vi "manuele bediening.vi"   [LabVIEW 2019]
uses:
  <vilib>/myRIO/Common/Instrument Driver Framework/Utilities/typedefs/Analog Scaling Constants.ctl
  <vilib>/myRIO/Common/Instrument Driver Framework/Utilities/typedefs/Analog Scaling Constants List.ctl
  <vilib>/myRIO/Common/Instrument Driver Framework/myRIO v1.0/AO/typedefs/AO Channels Enum.ctl
  <vilib>/myRIO/Common/Instrument Driver Framework/myRIO v1.0/AO/typedefs/AO Channels List.ctl
  <vilib>/myRIO/Common/Instrument Driver Framework/Utilities/typedefs/Generic FPGA Reference.ctl
  <vilib>/myRIO/Common/Instrument Driver Framework/Utilities/typedefs/myRIO v1.0 Reference.ctl
  <vilib>/myRIO/Common/Instrument Driver Framework/Utilities/typedefs/Hardware Version Enum.ctl
  <vilib>/myRIO/Common/Instrument Driver Framework/Utilities/typedefs/myRIO Generic Hardware Reference.ctl
  <vilib>/myRIO/Instrument Drivers/Onboard IO/AO/typedefs/AO Reference.ctl
  <vilib>/myRIO/Instrument Drivers/Onboard IO/AO/AO.lvlib
  <vilib>/myRIO/Instrument Drivers/Onboard IO/AO/vis/Write.vi
  <vilib>/userDefined/High Color/nirio_resource_hc.ctl
  <vilib>/myRIO/Common/Instrument Driver Framework/myRIO v1.0/AO/vis/myRIO v1.1 Open AO.vi
  <vilib>/myRIO/Instrument Drivers/Onboard IO/AO/vis/myRIO AO Open.xnode
  <vilib>/myRIO/Common/Instrument Driver Framework/Utilities/vis/Is FPGA Ref Available.vi
  <vilib>/myRIO/Express VI/Onboard IO/AO/AO Express VI.xnode
  interface.vi
types:
  T1 = typedef "AO.lvlib/AO Reference.ctl" = cluster{"myRIO Reference":T2, "AO Channel List":T6, "AO Scaling Constant List":T8}
  T2 = typedef "myRIO Generic Hardware Reference.ctl" = cluster{"myRIO Model":T3, "myRIO Hardware Reference":T4}
  T3 = typedef "Hardware Version Enum.ctl" = enum16{"Unknown", "myRIO-1900", "myRIO-1950", "roboRIO", "NI ELVIS RIO CM", "ELVIS III"}
  T4 = typedef "myRIO v1.0 Reference.ctl" = cluster{"Generic FPGA Reference":T5, "Allow multiple opens":bool}
  T5 = typedef "Generic FPGA Reference.ctl" = refnum<k20>
  T6 = typedef "AO Channels List.ctl" = T7[]
  T7 = typedef "AO Channels Enum.ctl" = enum16{"Not Connected", "AudioOut/Left", "AudioOut/Right", "C/AO0", "C/AO1", "A/AO0", "A/AO1", "B/AO0", "B/AO1"}
  T8 = typedef "Analog Scaling Constants List.ctl" = T9[]
  T9 = typedef "Analog Scaling Constants.ctl" = cluster{"LSB Weight (Volts)":dbl, "Offset (Volts)":dbl, "Signed?":bool}
  T10 = typedef "nirio_resource_hc.ctl" = tag
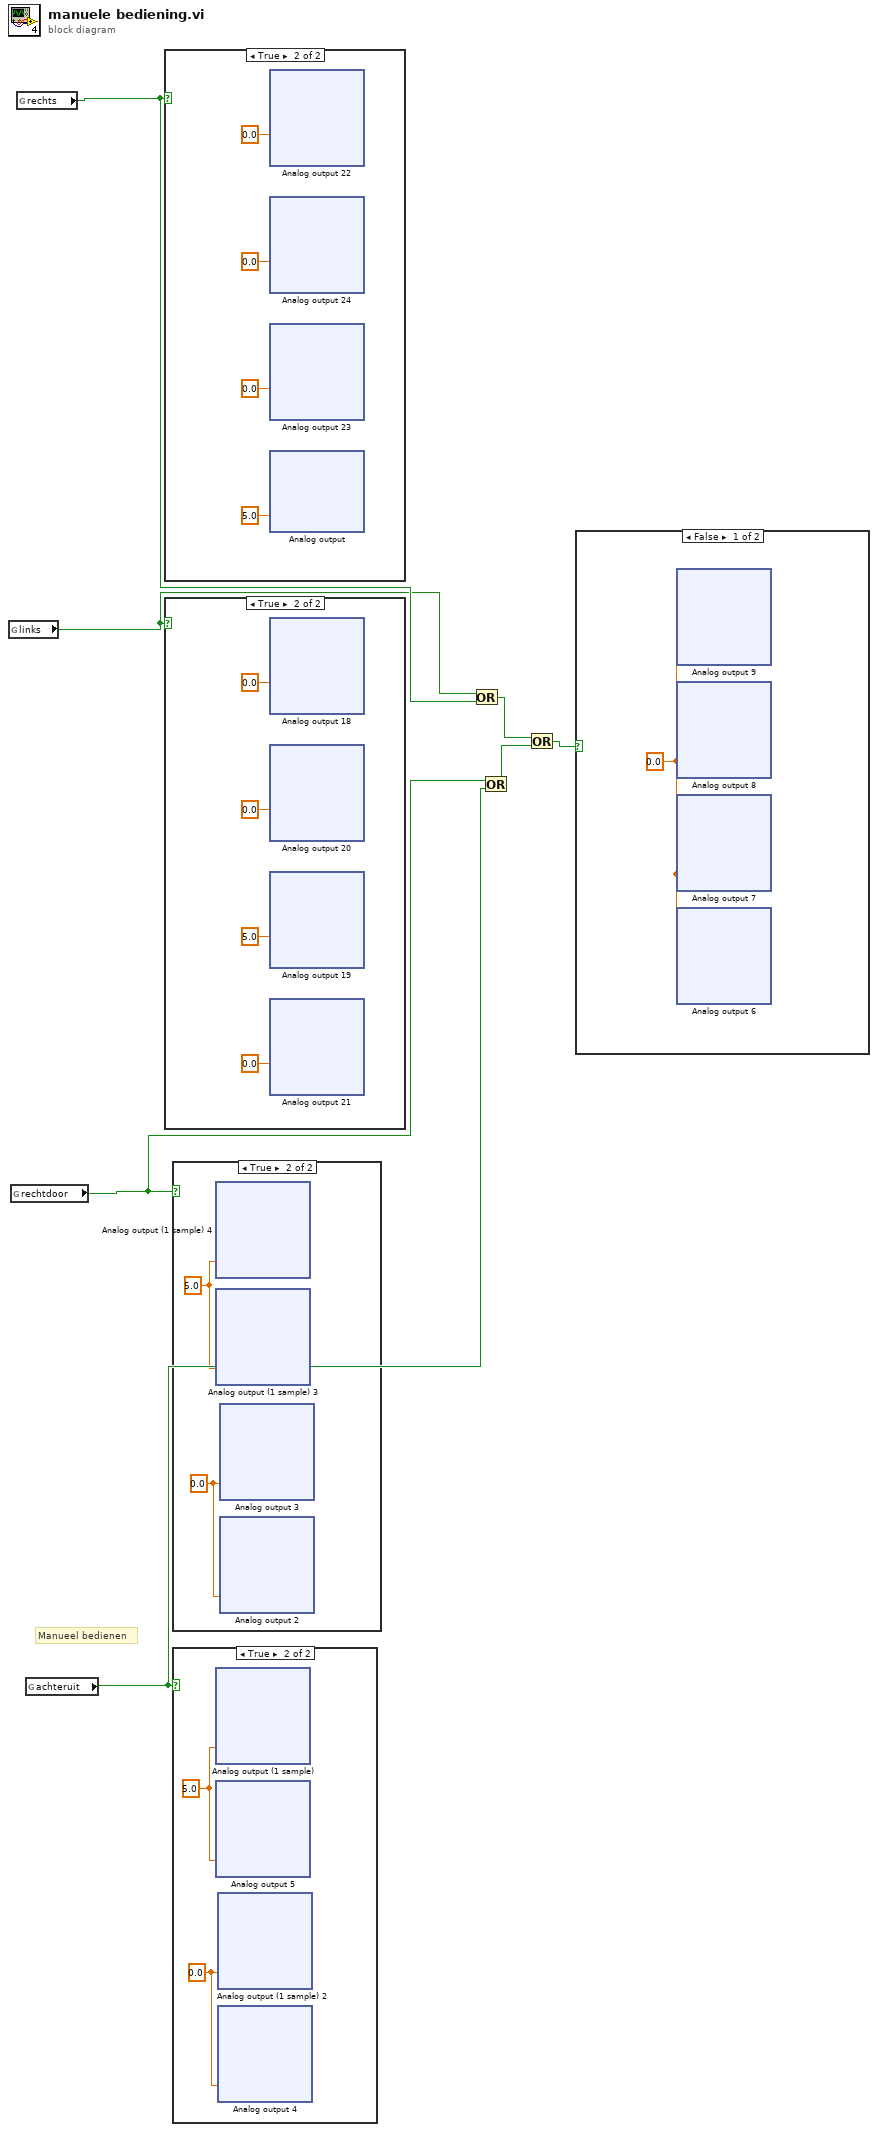
[diagram p0: block diagram]
diagram:
  # "Manueel bedienen"
  n1 = global read "interface.vi" "links"() -> (w3:bool)
  n2 = global read "interface.vi" "rechtdoor"() -> (w2:bool)
  n3 = global read "interface.vi" "rechts"() -> (w4:bool)
  n4 = global read "interface.vi" "achteruit"() -> (w1:bool)
  n5 = case shown="True" w4 {
    frame False {
    }
    frame True {
      n6 = xnode "Analog output 22"("B/AO1 (Pin 4)"=0.0) -> ()  [unwired: 1 in, 1 out]
      n7 = xnode "Analog output 24"("A/AO1 (Pin 4)"=0.0) -> ()  [unwired: 1 in, 1 out]
      n8 = xnode "Analog output 23"("B/AO0 (Pin 2)"=0.0) -> ()  [unwired: 1 in, 1 out]
      n9 = xnode "Analog output"("A/AO0 (Pin 2)"=5.0) -> ()  [unwired: 1 in, 1 out]
    }
  }
  n10 = case shown="True" w3 {
    frame False {
    }
    frame True {
      n11 = xnode "Analog output 18"("B/AO1 (Pin 4)"=0.0) -> ()  [unwired: 1 in, 1 out]
      n12 = xnode "Analog output 20"("A/AO1 (Pin 4)"=0.0) -> ()  [unwired: 1 in, 1 out]
      n13 = xnode "Analog output 19"("B/AO0 (Pin 2)"=5.0) -> ()  [unwired: 1 in, 1 out]
      n14 = xnode "Analog output 21"("A/AO0 (Pin 2)"=0.0) -> ()  [unwired: 1 in, 1 out]
    }
  }
  n15 = case shown="True" w2 {
    frame False {
    }
    frame True {
      w312 = 5.0
      w313 = 0.0
      n16 = xnode "Analog output (1 sample) 4"("A/AO0 (Pin 2)"=w312) -> ()  [unwired: 1 in, 1 out]
      n17 = xnode "Analog output (1 sample) 3"("B/AO0 (Pin 2)"=w312) -> ()  [unwired: 1 in, 1 out]
      n18 = xnode "Analog output 3"("A/AO1 (Pin 4)"=w313) -> ()  [unwired: 1 in, 1 out]
      n19 = xnode "Analog output 2"("B/AO1 (Pin 4)"=w313) -> ()  [unwired: 1 in, 1 out]
    }
  }
  n20 = case shown="True" w1 {
    frame False {
    }
    frame True {
      w462 = 5.0
      w463 = 0.0
      n21 = xnode "Analog output (1 sample)"("A/AO1 (Pin 4)"=w462) -> ()  [unwired: 1 in, 1 out]
      n22 = xnode "Analog output 5"("B/AO1 (Pin 4)"=w462) -> ()  [unwired: 1 in, 1 out]
      n23 = xnode "Analog output (1 sample) 2"("A/AO0 (Pin 2)"=w463) -> ()  [unwired: 1 in, 1 out]
      n24 = xnode "Analog output 4"("B/AO0 (Pin 2)"=w463) -> ()  [unwired: 1 in, 1 out]
    }
  }
  n25 = Or(x=w3, y=w4) -> (x .or. y?=w6:bool)
  n26 = Or(x=w2, y=w1) -> (x .or. y?=w7:bool)
  n27 = Or(x=w6, y=w7) -> (x .or. y?=w5:bool)
  n28 = case shown="False" w5 {
    frame False {
      w612 = 0.0
      n29 = xnode "Analog output 9"("A/AO0 (Pin 2)"=w612) -> ()  [unwired: 1 in, 1 out]
      n30 = xnode "Analog output 8"("A/AO1 (Pin 4)"=w612) -> ()  [unwired: 1 in, 1 out]
      n31 = xnode "Analog output 7"("B/AO0 (Pin 2)"=w612) -> ()  [unwired: 1 in, 1 out]
      n32 = xnode "Analog output 6"("B/AO1 (Pin 4)"=w612) -> ()  [unwired: 1 in, 1 out]
    }
    frame True {
    }
  }
